vi "Write RM DMA.vi"(4 "Iteration":i32, 8 "error in":errorcluster, 9 "VMIC reference in":T2, 10 "Block descriptors":T1[](array[typedef]), 11 "Values":dbl[](array[numeric])) -> (0 "error out":errorcluster, 1 "VMIC reference out":T2, 2 "Write Duration":u32, 3 "Values":dbl[](array[numeric]))   [LabVIEW 2015, in "RefMem DMA Custom Device.lvlib"]
uses:
  RefMem DMA Custom Device.lvlib
  Block descriptor.ctl
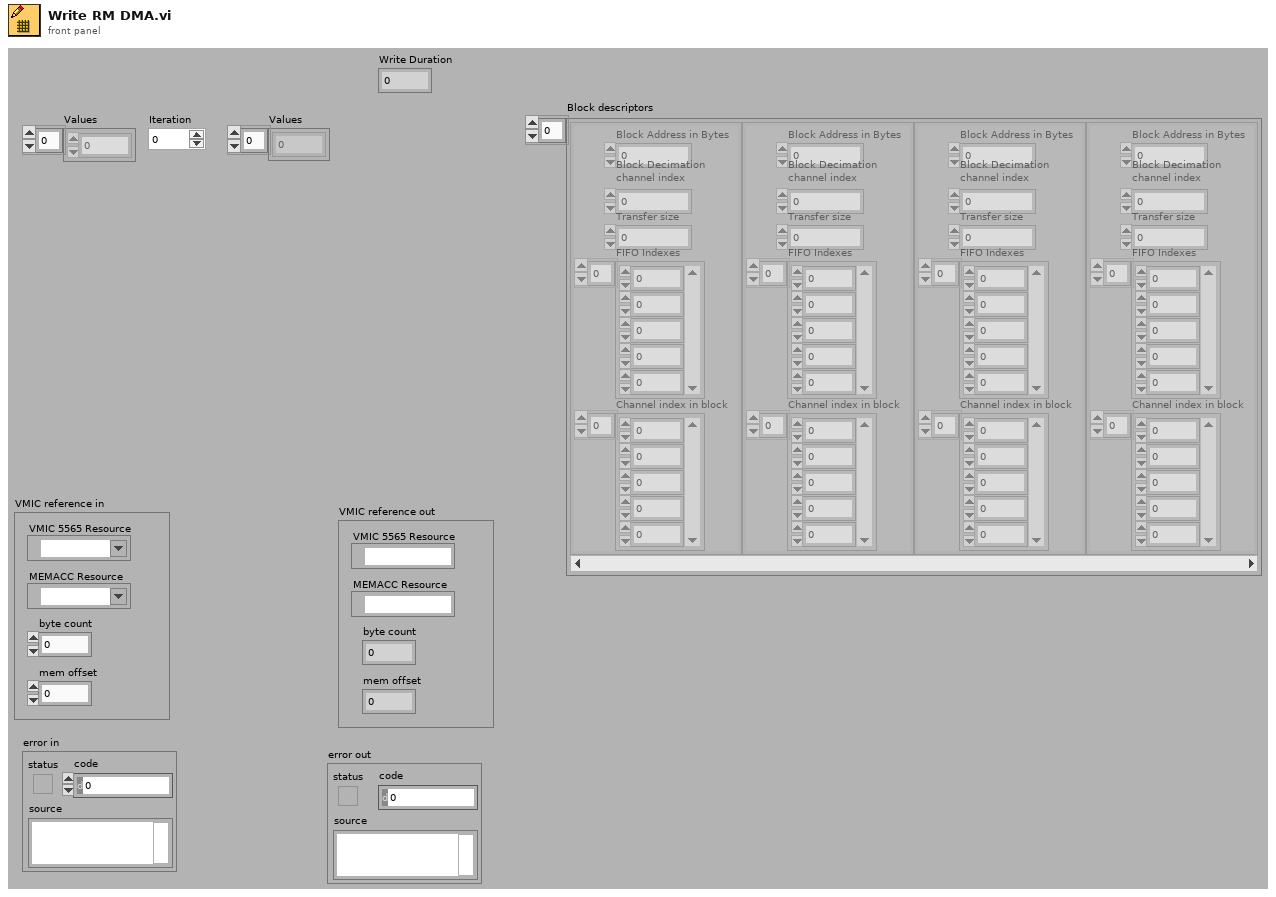
[diagram p1: front panel]
types:
  T1 = typedef "RefMem DMA Custom Device.lvlib/Block descriptor.ctl" = cluster{"Block Address in Bytes":u32, "Block Decimation \nchannel index":i32, "Transfer size":u32, "FIFO Indexes":i32[], "Channel index in block":i32[]}
  T2 = cluster{"VMIC 5565 Resource":refnum<visa-resource-name>, "MEMACC Resource":refnum<visa-resource-name>, "byte count":u32, "mem offset":u32}
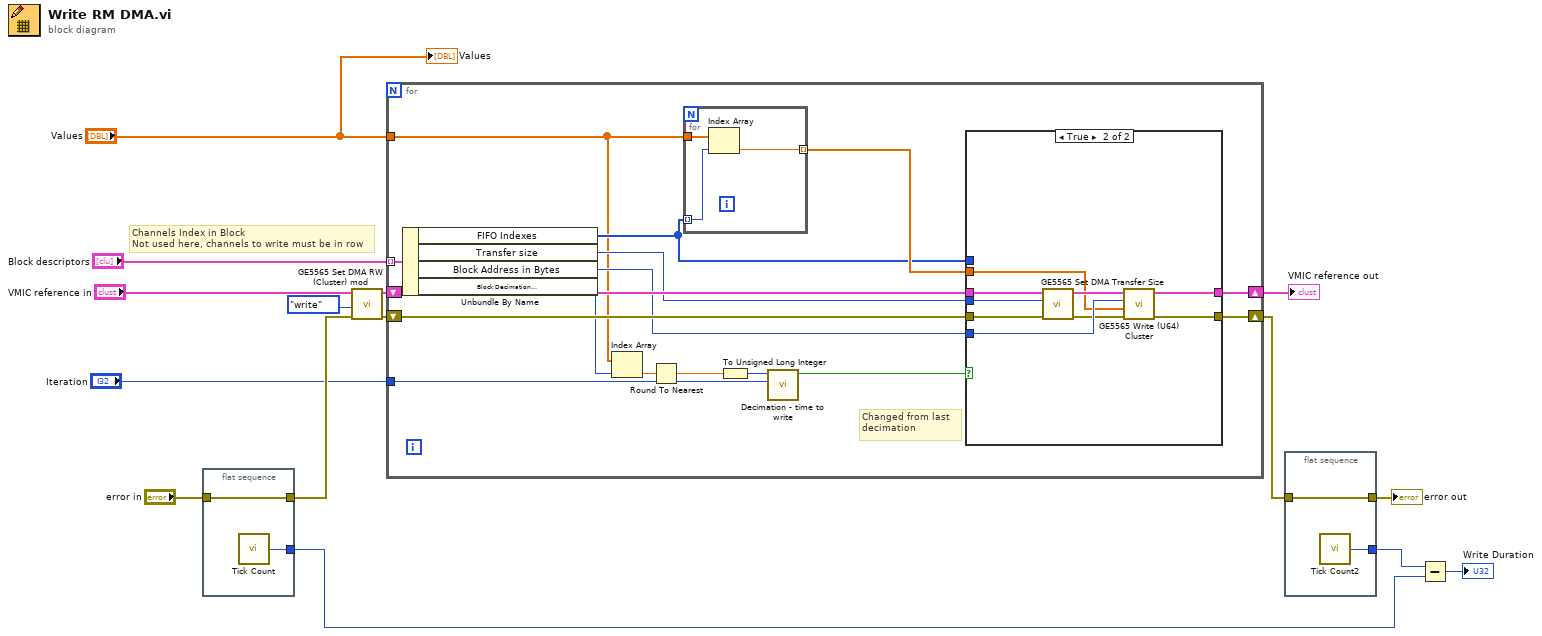
[diagram p0: block diagram]
diagram:
  # "Channels Index in Block\nNot used here, channels to write must be in row"
  n1 = flat-sequence {
    tunnel: [w17] -> w5
    tunnel: "error in" -> [w17]
    tunnel: [w16] -> w11
    frame #0 {
      n2 = call "Tick Count"() -> ("Tick Count(uSec)"=w16:u32)
    }
  }
  n3 = call "GE5565 Set DMA RW (Cluster) mod.vi"("error in (no error)"=w5, "operation (read)"=enum16{"read", "write"}."write", "VMIC-5565"="VMIC reference in") -> ("error out"=w4:errorcluster, "VMIC-5565"=w6:T2)  [unwired: 3 in]
  n4 = for "Write Output Values to System" {
    shift-right: [w30] -> w14
    shift-left: w4 -> [w29]
    tunnel: "Values" -> [w23]
    shift-right: [w33] -> w3
    shift-left: w6 -> [w31]
    tunnel: "Iteration" -> [w32]
    tunnel: "Block descriptors" -> [w28] mode=indexing
    # "Changed from last\ndecimation"
    n5 = Unbundle By Name(w28) -> ("FIFO Indexes"=w24:i32[], "Transfer size"=w26:u32, "Block Address in Bytes"=w27:u32, "Block Decimation \nchannel index"=w22:i32)
    n6 = Index Array(array=w23, index=w22) -> (element=w21:dbl)
    n7 = Round To Nearest(number=w21) -> (nearest integer value=w20:dbl)
    n8 = for {
      tunnel: w24 -> [w34] mode=indexing
      tunnel: w23 -> [w36]
      tunnel: [w35] -> w25 mode=indexing
      n9 = Index Array(array=w36, index=w34) -> (element=w35:dbl)
    }
    n10 = To Unsigned Long Integer(number=w20) -> (unsigned 32bit integer=w19:u32)
    n11 = call "Decimation - time to write.vi"("Iteration"=w32, "Decimation"=w19) -> ("Ready"=w18:bool)  [unwired: 9 in]
    n12 = case shown="True" w18 {
      tunnel: [w37 w47] -> w30
      tunnel: [w38 w46] -> w33
      tunnel: w29 -> [w37 w45]
      tunnel: w31 -> [w38 w44]
      tunnel: w26 -> [_ w43]
      tunnel: w27 -> [_ w42]
      tunnel: w25 -> [_ w39]
      tunnel: w24 -> [_ _]
      frame False {
      }
      frame True {
        n13 = call "GE5565 Set DMA Transfer Size.vi"("error in (no error)"=w45, "Transfer Size"=w43, "VMIC-5565"=w44) -> ("error out"=w40:errorcluster, "VMIC-5565"=w41:T2)  [unwired: 3 in]
        n14 = call "GE5565 Write (U64) Cluster.vi"("error in (no error)"=w40, "buffer"=w39, "offset (0)"=w42, "VMIC reference in"=w41) -> ("error out"=w47:errorcluster, "VMIC reference out"=w46:T2)  [unwired: 6 in]
      }
    }
  }
  "VMIC reference out" <- w3
  n15 = flat-sequence {
    tunnel: [w49] -> w13
    tunnel: w14 -> [w49]
    tunnel: [w48] -> w12
    frame #0 {
      n16 = call "Tick Count2"() -> ("Tick Count(uSec)"=w48:u32)
    }
  }
  n17 = Subtract(x=w12, y=w11) -> (x-y=→"Write Duration":u32)
  "Values" <- "Values"
  "error out" <- w13
